vi "Clean (After).vi"() -> ()   [LabVIEW 2010]
doc: "A sample VI demonstrating a cleaned up front panel and block diagram."
panel:
  in  "Math Functions":enum32{"Add", "Multiply"}(tab)
  in  "Num 1":dbl
  in  "Num 2":dbl
  out "Result":dbl
  in  "Num 1":dbl
  in  "Num 2":dbl
  out "Result":dbl
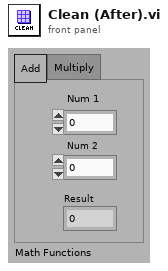
[diagram p1: front panel]
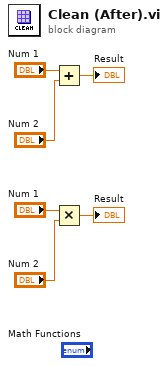
[diagram p0: block diagram]
diagram:
  n1 = Add(x="Num 1", y="Num 2") -> (x+y=→"Result":dbl)
  n2 = Multiply(x="Num 1", y="Num 2") -> (x*y=→"Result":dbl)
